vi "Sub_Preprocessing_FEA_Moment_of_Inertia.vi"(10 "Height":dbl, 11 "Width":dbl) -> (3 "Numeric":dbl)   [LabVIEW 2021]
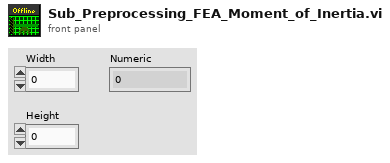
[diagram p1: front panel]
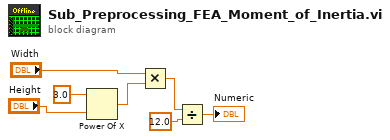
[diagram p0: block diagram]
diagram:
  n1 = Power Of X(1:"Height", 2:3.0 ("x")) -> (0:w4:dbl)
  n2 = Multiply(x="Width", y=w4) -> (x*y=w5:dbl)
  n3 = Divide(x=w5, y=12.0) -> (x/y=→"Numeric":dbl)
